vi "VisionExecute.v.vi"   [LabVIEW 2020]
uses:
  <vilib>/Rock Robotics/WPI/ThirdParty/JAS_Junk/TrajLib/Trajectory_Library.lvlib
  <vilib>/Rock Robotics/WPI/ThirdParty/PhotonVisionLib/PhotonVisionLib.lvlib
  <vilib>/Rock Robotics/WPI/ThirdParty/PhotonPoseStrategy_ENUM.ctl
  VisionGlobal.vi
  <vilib>/Rock Robotics/WPI/ThirdParty/JAS_Junk/TrajLib/TypeDef/TRANSLATION2D.ctl
  <vilib>/Rock Robotics/WPI/ThirdParty/JAS_Junk/TrajLib/TypeDef/ROTATION2D.ctl
  <vilib>/Rock Robotics/WPI/ThirdParty/JAS_Junk/TrajLib/TypeDef/POSE2D.ctl
types:
  T1 = typedef "PhotonVisionLib.lvlib/PhotonPoseStrategy_ENUM.ctl" = enum16{"LOWEST_AMBIGUITY", "CLOSEST_TO_CAMERA_HEIGHT", "CLOSEST_TO_REFERENCE_POSE", "CLOSEST_TO_LAST_POSE", "AVERAGE_BEST_TARGETS"}
  T2 = typedef "Trajectory_Library.lvlib/TRANSLATION3D.ctl" = cluster{"X":dbl, "Y":dbl, "Z":dbl}
  T3 = typedef "Trajectory_Library.lvlib/ROTATION3D.ctl" = cluster{"Q_quaternion":T4}
  T4 = typedef "Trajectory_Library.lvlib/QUATERNION.ctl" = cluster{"R":dbl, "V":dbl[]}
  T5 = typedef "Trajectory_Library.lvlib/TRANSFORM3D.ctl" = cluster{"TRANSLATION3D":T2, "ROTATION3D":T3, "XF":bool}
  T6 = typedef "PhotonVisionLib.lvlib/PhotonPipelineResultType.ctl" = cluster{"TargetCount":i32, "Latency_MilliSec":dbl, "Targets":T7[], "TimeStampSec":dbl}
  T7 = typedef "PhotonVisionLib.lvlib/PhotonTrackedTargetType.ctl" = cluster{"Yaw":dbl, "Pitch":dbl, "Area":dbl, "Skew":dbl, "MinAreaRectCorners":T8[], "BestCameraToTarget":T5, "FiiducialId":i32, "AltCameraToTarget":T5, "PoseAmbiguity":dbl, "DetectedCorners":T8[]}
  T8 = typedef "PhotonVisionLib.lvlib/TargetCornerType.ctl" = cluster{"X":dbl, "Y":dbl}
  T9 = typedef "PhotonVisionLib.lvlib/PhotonPoseEstimator_Configuration.ctl" = cluster{"Strategy":T1, "Camera":string, "Initial Pose":T10, "AprilTagField":enum16{"2022 Rapid React", "2023 Charged Up"}, "HighestAmbiguity":dbl, "Use Custom Field":bool, "Custom AprilTag Field":T11, "RobotToCamera":T5}
  T10 = typedef "Trajectory_Library.lvlib/POSE3D.ctl" = cluster{"Translation3d":T2, "Rotation3d":T3}
  T11 = typedef "Trajectory_Library.lvlib/AprilTagFieldLayout.ctl" = cluster{"AprilTagMap":map{i32, T12}, "FieldLength":dbl, "FieldWidth":dbl, "OriginPosition ":T13, "OriginPose3d":T10}
  T12 = typedef "Trajectory_Library.lvlib/AprilTag.ctl" = cluster{"ID":i32, "POSE3D":T10}
  T13 = typedef "Trajectory_Library.lvlib/AprilTagFieldLayoutOrignPosition_ENUM.ctl" = enum16{"kBlueAllianceWallRightSide,", "kRedAllianceWallRightSide,"}
  T14 = typedef "PhotonVisionLib.lvlib/PhotonEstimatedRobotPoseType.ctl" = cluster{"EstimatedPose":T10, "TimeStamp_Seconds":dbl}
  T15 = typedef "Trajectory_Library.lvlib/POSE2D.ctl" = cluster{"TRANSLATION":T16, "ROTATION":T17}
  T16 = typedef "Trajectory_Library.lvlib/TRANSLATION2D.ctl" = cluster{"X":dbl, "Y":dbl}
  T17 = typedef "Trajectory_Library.lvlib/ROTATION2D.ctl" = cluster{"VALUE":dbl, "COS":dbl, "SIN":dbl}
  T18 = typedef "Trajectory_Library.lvlib/SWERVE_DRIVE_KINEMATICS.ctl" = cluster{"NumModules":i32, "InverseKinematics":T19, "ForwardKinematics":T19, "Modules":T16[], "PrevCoR":T16, "SavedModuleStates":T20[]}
  T19 = typedef "NI_Matrix.lvlib/RealMatrix.ctl" = dbl[][]
  T20 = typedef "Trajectory_Library.lvlib/SWERVE_DRIVE_MODULE_STATE.ctl" = cluster{"Speed":dbl, "Angle":T17}
  T21 = typedef "Trajectory_Library.lvlib/SWERVE_DRIVE_MODULE_POSITION.ctl" = cluster{"Distance":dbl, "Angle":T17, "P":bool}
  T22 = typedef "Trajectory_Library.lvlib/SWERVE_DRIVE_POSE_EST2_CONFIG.ctl" = cluster{"Wheel_Locations M":T16[], "Odom X std dev M":dbl, "Odom Y std dev M":dbl, "Odom Heading std dev Rad":dbl, "Vision X std dev M":dbl, "Vision Y std dev M":dbl, "Vision Heading std dev Rad":dbl}
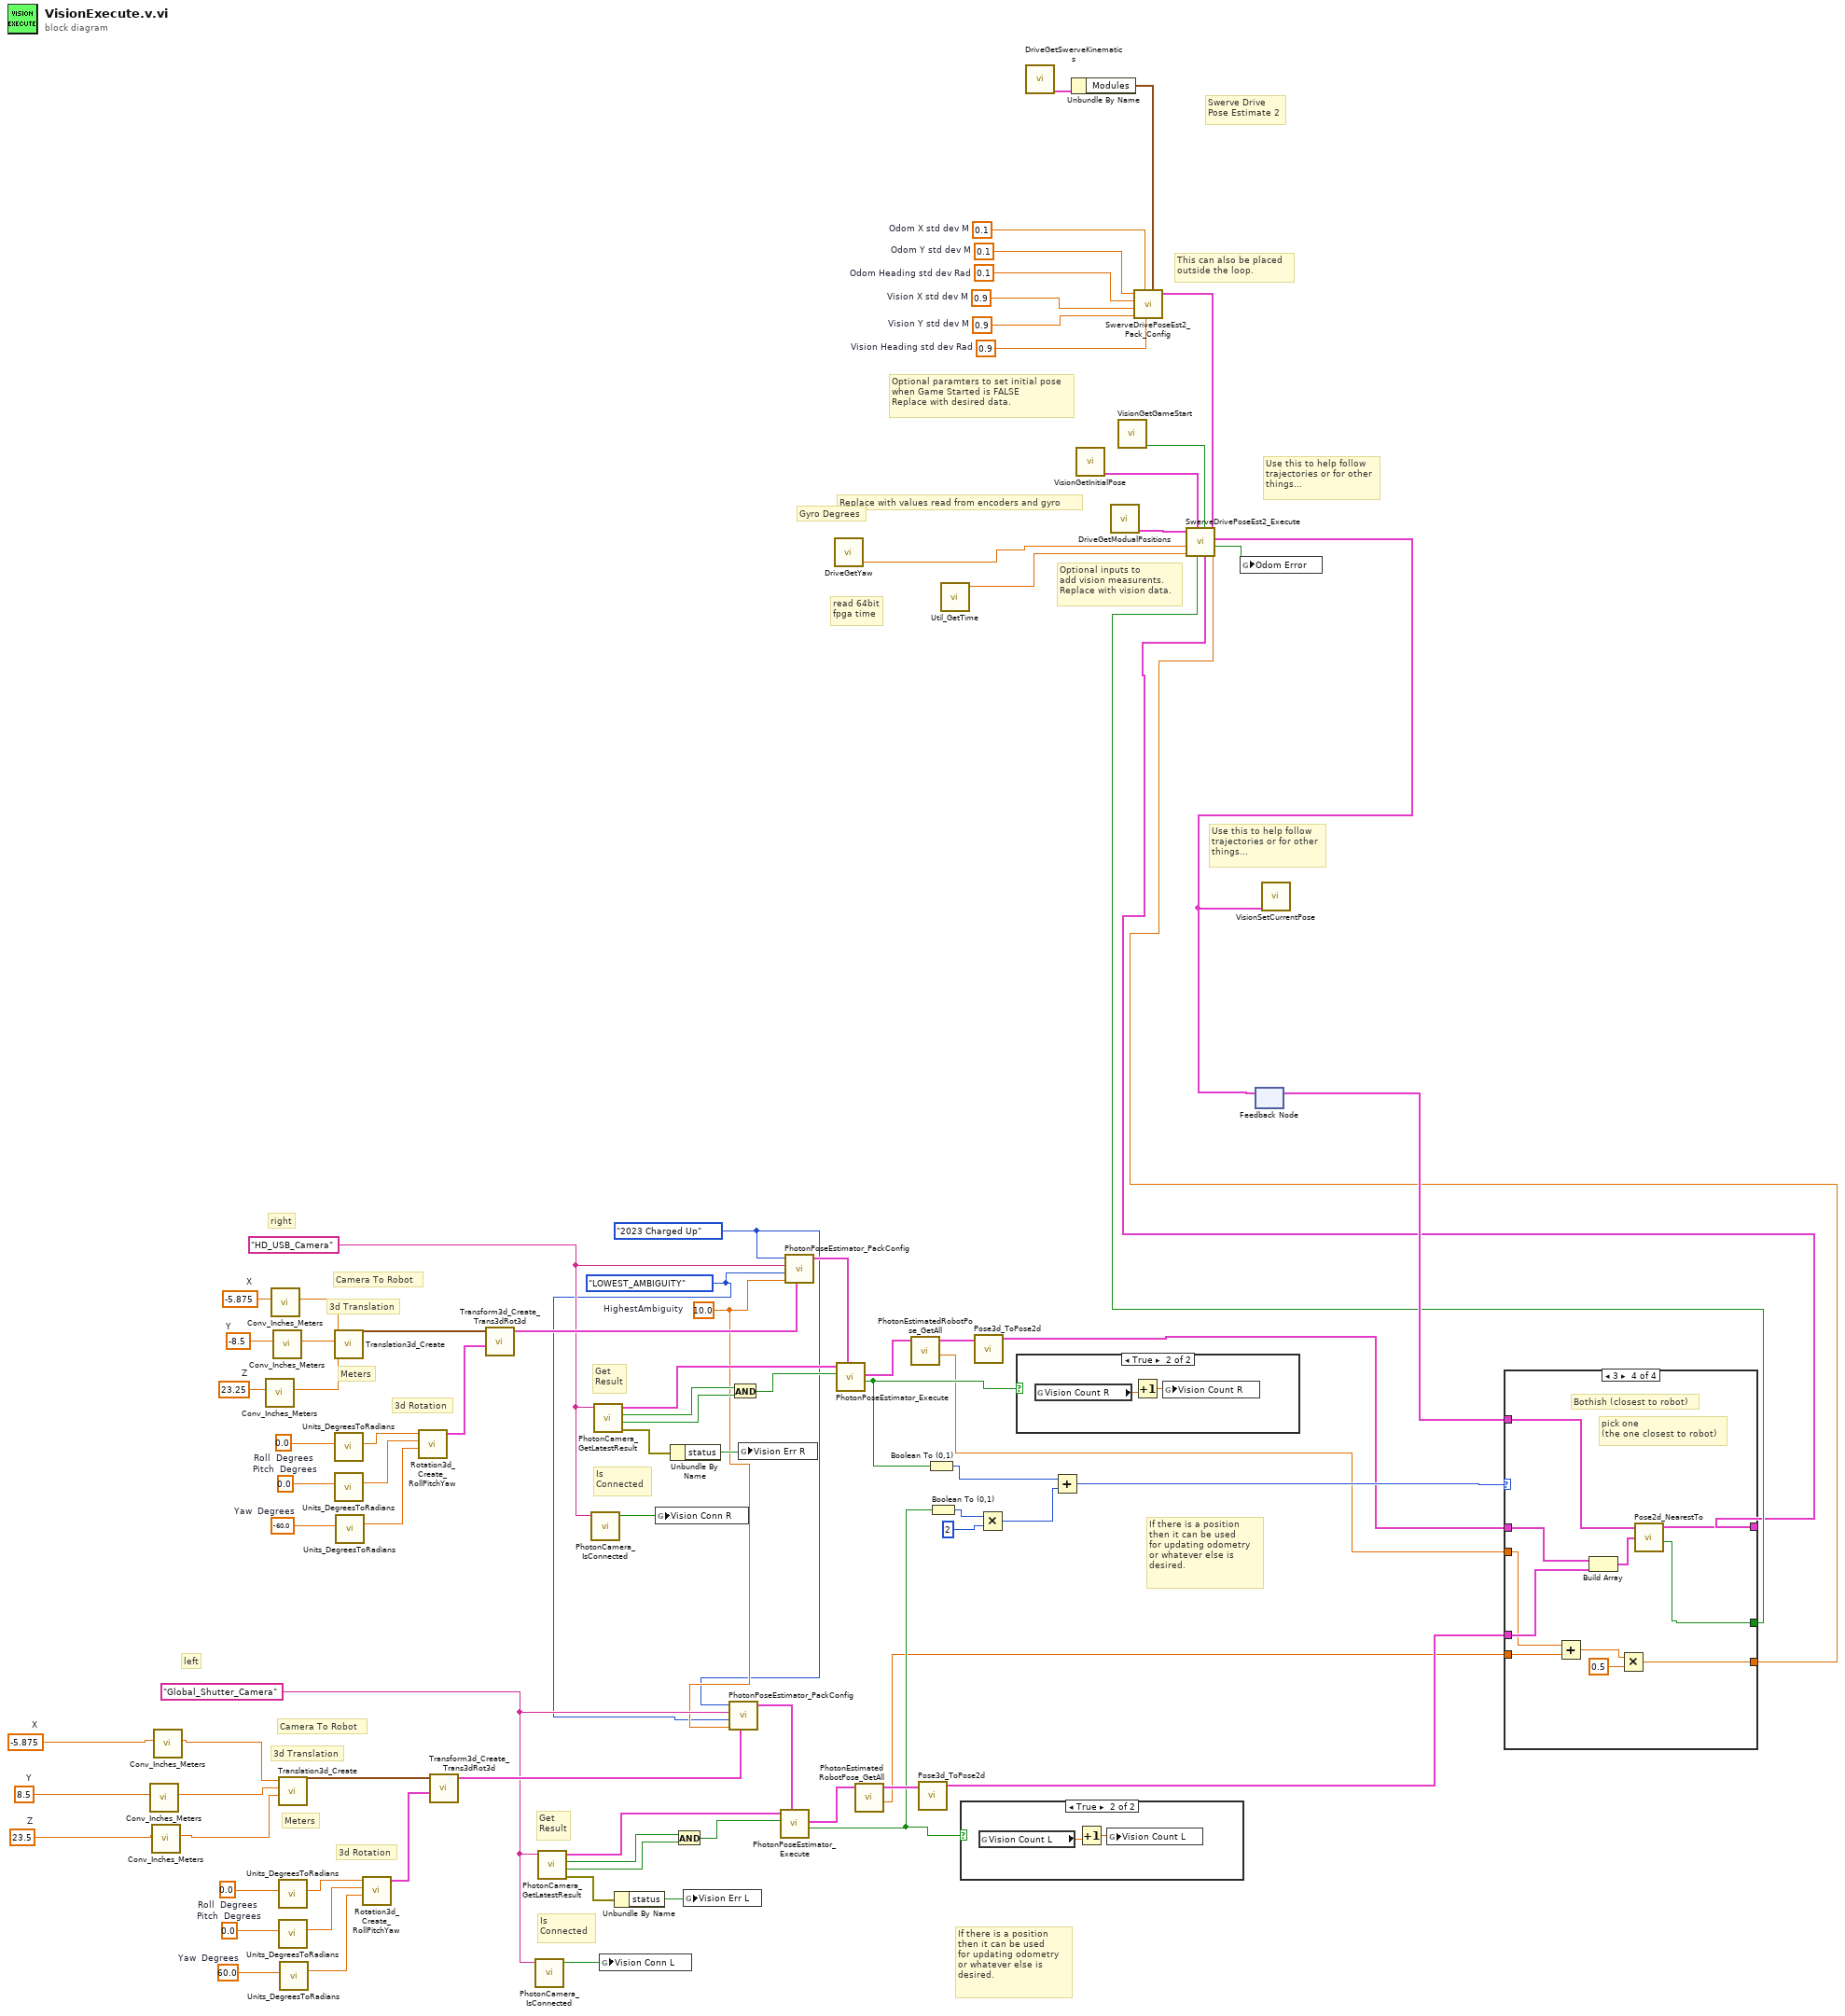
[diagram p0: block diagram]
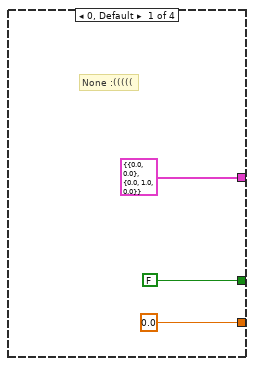
[diagram p2: hidden frame]
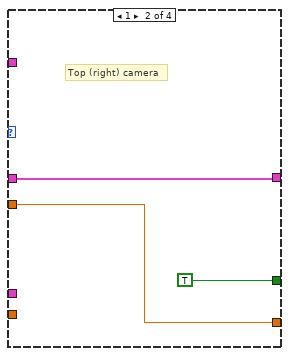
[diagram p3: hidden frame]
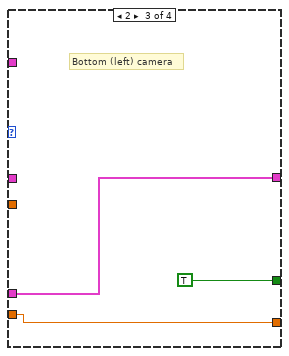
[diagram p4: hidden frame]
diagram:
  w14 = 0.1  # Odom Y std dev M
  w15 = 0.1  # Odom Heading std dev Rad
  w16 = 0.9  # Vision X std dev M
  w17 = 0.9  # Vision Y std dev M
  w18 = 0.1  # Odom X std dev M
  w19 = 0.9  # Vision Heading std dev Rad
  w59 = 0.0  # Roll  Degrees
  w58 = 0.0  # Pitch  Degrees
  w57 = 60.0  # Yaw  Degrees
  w42 = 23.5  # Z
  w46 = -5.875  # X
  w44 = 8.5  # Y
  w53 = "Global_Shutter_Camera" ("CameraName")
  w79 = 0.0  # Roll  Degrees
  w78 = 0.0  # Pitch  Degrees
  w77 = -60.0  # Yaw  Degrees
  w36 = 23.25  # Z
  w40 = -5.875  # X
  w38 = -8.5  # Y
  w34 = 10.0  # HighestAmbiguity
  w33 = PhotonPoseStrategy_ENUM."LOWEST_AMBIGUITY" ("Strategy")
  w32 = enum16{"2022 Rapid React", "2023 Charged Up"}."2023 Charged Up" ("AprilTagField")
  w73 = "HD_USB_Camera" ("CameraName")
  # "Optional inputs to\nadd vision measurents.\nReplace with vision data."
  # "Replace with values read from encoders and gyro"
  # "Optional paramters to set initial pose\nwhen Game Started is FALSE\nReplace with desired data."
  # "read 64bit\nfpga time"
  # "This can also be placed \noutside the loop."
  # "Use this to help follow\ntrajectories or for other\nthings..."
  # "Swerve Drive \nPose Estimate 2"
  # "Use this to help follow\ntrajectories or for other\nthings..."
  # "right"
  # "left"
  # "If there is a position\nthen it can be used\nfor updating odometry\nor whatever else is \ndesired."
  # "Meters"
  # "Camera To Robot"
  # "3d Rotation"
  # "3d Translation"
  # "Is\nConnected"
  # "Get\nResult"
  # "If there is a position\nthen it can be used\nfor updating odometry\nor whatever else is \ndesired."
  # "Meters"
  # "Camera To Robot"
  # "3d Rotation"
  # "3d Translation"
  # "Is\nConnected"
  # "Get\nResult"
  # "Gyro Degrees"
  n1 = call <vilib>:"Conv_Inches_Meters.vi"("INCH"=w44) -> ("Meters"=w43:dbl)  [unwired: 10 in]
  n2 = call <vilib>:"Conv_Inches_Meters.vi"("INCH"=w42) -> ("Meters"=w41:dbl)  [unwired: 10 in]
  n3 = call <vilib>:"Conv_Inches_Meters.vi"("INCH"=w46) -> ("Meters"=w45:dbl)  [unwired: 10 in]
  n4 = call <vilib>:"Conv_Inches_Meters.vi"("INCH"=w36) -> ("Meters"=w35:dbl)  [unwired: 10 in]
  n5 = call <vilib>:"Conv_Inches_Meters.vi"("INCH"=w40) -> ("Meters"=w39:dbl)  [unwired: 10 in]
  n6 = call <vilib>:"Conv_Inches_Meters.vi"("INCH"=w38) -> ("Meters"=w37:dbl)  [unwired: 10 in]
  n7 = call <vilib>:"Translation3d_Create.vi"("Z"=w41, "Y"=w43, "X"=w45) -> ("TRANSLATION3D"=w60:T2)  [unwired: 8 in]
  n8 = call <vilib>:"Units_DegreesToRadians.vi"("Degrees"=w59) -> ("Radians"=w56:dbl)  [unwired: 10 in]
  n9 = call <vilib>:"Units_DegreesToRadians.vi"("Degrees"=w58) -> ("Radians"=w55:dbl)  [unwired: 10 in]
  n10 = call <vilib>:"Units_DegreesToRadians.vi"("Degrees"=w57) -> ("Radians"=w54:dbl)  [unwired: 10 in]
  n11 = call <vilib>:"Translation3d_Create.vi"("Z"=w35, "Y"=w37, "X"=w39) -> ("TRANSLATION3D"=w80:T2)  [unwired: 8 in]
  n12 = call <vilib>:"Units_DegreesToRadians.vi"("Degrees"=w79) -> ("Radians"=w76:dbl)  [unwired: 10 in]
  n13 = call <vilib>:"Units_DegreesToRadians.vi"("Degrees"=w78) -> ("Radians"=w75:dbl)  [unwired: 10 in]
  n14 = call <vilib>:"Units_DegreesToRadians.vi"("Degrees"=w77) -> ("Radians"=w74:dbl)  [unwired: 10 in]
  n15 = call <vilib>:"Rotation3d_Create_RollPitchYaw.vi"("Yaw"=w54, "Pitch"=w55, "Roll"=w56) -> ("Rotation3d"=w61:T3)  [unwired: 8 in]
  n16 = call <vilib>:"Rotation3d_Create_RollPitchYaw.vi"("Yaw"=w74, "Pitch"=w75, "Roll"=w76) -> ("Rotation3d"=w81:T3)  [unwired: 8 in]
  n17 = call <vilib>:"Transform3d_Create_Trans3dRot3d.vi"("Rotation3d"=w61, "Translation3d"=w60) -> ("Transform3d"=w62:T5)  [unwired: 9 in]
  n18 = call <vilib>:"Transform3d_Create_Trans3dRot3d.vi"("Rotation3d"=w81, "Translation3d"=w80) -> ("Transform3d"=w82:T5)  [unwired: 9 in]
  n19 = call <vilib>:"PhotonCamera_IsConnected.vi"("CameraName"=w53) -> ("IsConnected"=w49:bool)  [unwired: 9 in, 1 out]
  n20 = call <vilib>:"PhotonCamera_GetLatestResult.vi"("CameraName"=w53) -> ("error out"=w48:errorcluster, "New Data"=w66:bool, "HasTargets"=w65:bool, "PipelineResult"=w63:T6)  [unwired: 7 in]
  n21 = call <vilib>:"PhotonCamera_IsConnected.vi"("CameraName"=w73) -> ("IsConnected"=w69:bool)  [unwired: 9 in, 1 out]
  n22 = call <vilib>:"PhotonCamera_GetLatestResult.vi"("CameraName"=w73) -> ("error out"=w68:errorcluster, "New Data"=w86:bool, "HasTargets"=w85:bool, "PipelineResult"=w83:T6)  [unwired: 7 in]
  n23 = global write "VisionGlobal.vi" "Vision Conn L"(w49) -> ()
  n24 = Unbundle By Name(w48) -> ("status"=w47:bool)
  n25 = global write "VisionGlobal.vi" "Vision Conn R"(w69) -> ()
  n26 = Unbundle By Name(w68) -> ("status"=w67:bool)
  n27 = And(x=w65, y=w66) -> (x .and. y?=w64:bool)
  n28 = global write "VisionGlobal.vi" "Vision Err L"(w47) -> ()
  n29 = call <vilib>:"PhotonPoseEstimator_PackConfig.vi"("RobotToCamera"=w62, "HighestAmbiguity"=w34, "Strategy"=w33, "Camera"=w53, "AprilTagField"=w32) -> ("PoseEstimator_Configuration"=w52:T9)  [unwired: 6 in]
  n30 = And(x=w85, y=w86) -> (x .and. y?=w84:bool)
  n31 = global write "VisionGlobal.vi" "Vision Err R"(w67) -> ()
  n32 = call <vilib>:"PhotonPoseEstimator_Execute.vi"("Configuration"=w52, "PIpeline Has \nNew Results"=w64, "PipelineResult"=w63) -> ("Pos Found"=w30:bool, "PhotonEstimatedRobotPose"=w51:T14)  [unwired: 6 in, 1 out]
  n33 = call <vilib>:"PhotonPoseEstimator_PackConfig.vi"("RobotToCamera"=w82, "HighestAmbiguity"=w34, "Strategy"=w33, "Camera"=w73, "AprilTagField"=w32) -> ("PoseEstimator_Configuration"=w72:T9)  [unwired: 6 in]
  n34 = call "DriveGetYaw.vi"() -> ("Yaw"=w9:dbl)  [unwired: 11 in]
  n35 = call <vilib>:"PhotonPoseEstimator_Execute.vi"("Configuration"=w72, "PIpeline Has \nNew Results"=w84, "PipelineResult"=w83) -> ("Pos Found"=w31:bool, "PhotonEstimatedRobotPose"=w71:T14)  [unwired: 6 in, 1 out]
  n36 = call <vilib>:"PhotonEstimatedRobotPose_GetAll.vi"("PhotonEstimatedRobotPose"=w51) -> ("TimeStamp_Seconds"=w20:dbl, "EstimatedPose"=w50:T10)  [unwired: 9 in]
  n37 = call <vilib>:"PhotonEstimatedRobotPose_GetAll.vi"("PhotonEstimatedRobotPose"=w71) -> ("TimeStamp_Seconds"=w21:dbl, "EstimatedPose"=w70:T10)  [unwired: 9 in]
  n38 = call <vilib>:"Pose3d_ToPose2d.vi"("in Pose3d"=w50) -> ("out Pose2d"=w23:T15)  [unwired: 10 in]
  n39 = Boolean To (0,1)(Boolean=w31) -> (0, 1=w26:i16)
  n40 = Boolean To (0,1)(Boolean=w30) -> (0, 1=w29:i16)
  n41 = call <vilib>:"Util_GetTime.vi"() -> ("FPGA_Time_Seconds"=w6:dbl)  [unwired: 9 in, 2 out]
  n42 = case shown="True" w30 {
    frame False {
    }
    frame True {
      n43 = global read "VisionGlobal.vi" "Vision Count L"() -> (w87:dbl)
      n44 = Increment(x=w87) -> (x+1=w88:dbl)
      n45 = global write "VisionGlobal.vi" "Vision Count L"(w88) -> ()
    }
  }
  n46 = call <vilib>:"Pose3d_ToPose2d.vi"("in Pose3d"=w70) -> ("out Pose2d"=w24:T15)  [unwired: 10 in]
  n47 = Multiply(x=w29, y=i16 2) -> (x*y=w27:i16)
  n48 = case shown="True" w31 {
    frame False {
    }
    frame True {
      n49 = global read "VisionGlobal.vi" "Vision Count R"() -> (w89:dbl)
      n50 = Increment(x=w89) -> (x+1=w90:dbl)
      n51 = global write "VisionGlobal.vi" "Vision Count R"(w90) -> ()
    }
  }
  n52 = call "DriveGetSwerveKinematics.vi"() -> ("SWERVE_DRIVE_KINEMATICS"=w2:T18)  [unwired: 11 in]
  n53 = Add(x=w26, y=w27) -> (x+y=w25:i16)
  n54 = Unbundle By Name(w2) -> ("Modules"=w1:T16[])
  n55 = call "VisionGetInitialPose.vi"() -> ("InitialPose"=w7:T15)  [unwired: 10 in]
  n56 = call "DriveGetModualPositions.vi"() -> ("Swerve_Drive_Modual_Position"=w10:T21[])  [unwired: 11 in]
  n57 = call "VisionGetGameStart.vi"() -> ("Game Start"=w8:bool)  [unwired: 11 in]
  n58 = call <vilib>:"SwerveDrivePoseEst2_Pack_Config.vi"("Wheel_Locations M"=w1, "Vision Heading std dev Rad"=w19, "Odom X std dev M"=w18, "Vision Y std dev M"=w17, "Vision X std dev M"=w16, "Odom Heading std dev Rad"=w15, "Odom Y std dev M"=w14) -> ("SwervePoseEst2Config"=w13:T22)  [unwired: 4 in]
  n59 = feedback #1() -> (w22:T15)  [unwired: 1 in]
  n60 = case shown="3" w25 {
    tunnel: w24 -> [_ w95 _ w108]
    tunnel: w23 -> [_ _ w98 w107]
    tunnel: w22 -> [_ _ _ w109]
    tunnel: [FALSE ("Found") TRUE ("Found") TRUE ("Found") w105] -> w5
    tunnel: w21 -> [_ w96 _ w104]
    tunnel: w20 -> [_ _ w99 w103]
    tunnel: [T15 {"TRANSLATION"={"X"=0.0, "Y"=0.0}, "ROTATION"={"VALUE"=0.0, "COS"=1.0, "SIN"=0.0}} ("Nearest Pose") w95 w98 w106] -> w4
    tunnel: [0.0 w96 w99 w100] -> w3
    frame 0, Default {
      # "None :((((("
    }
    frame 1 {
      # "Top (right) camera"
    }
    frame 2 {
      # "Bottom (left) camera"
    }
    frame 3 {
      # "pick one \n(the one closest to robot)"
      # "Bothish (closest to robot)"
      n61 = Add(x=w104, y=w103) -> (x+y=w102:dbl)
      n62 = Build Array(w108, w107) -> (w110:T15[])
      n63 = Multiply(x=w102, y=0.5) -> (x*y=w100:dbl)
      n64 = call <vilib>:"Pose2d_NearestTo.vi"("other POSE"=w110, "in POSE"=w109) -> ("Found"=w105:bool, "Nearest Pose"=w106:T15)  [unwired: 8 in]
    }
  }
  n65 = call <vilib>:"SwerveDrivePoseEst2_Execute.vi"("Vision TImeStamp_Seconds"=w3, "SwervePoseEst2Config"=w13, "visionRobotPose"=w4, "Game Started"=w8, "Add Vision Meas"=w5, "InitialPose"=w7, "Pass Through Time"=w6, "Gyro Degrees"=w9, "Module Positions"=w10) -> ("Error"=w11:bool, "Estimated Pose"=w12:T15)  [unwired: 1 in]
  n66 = global write "VisionGlobal.vi" "Odom Error"(w11) -> ()
  n67 = feedback-in #1(w12) -> ()
  n68 = call "VisionSetCurrentPose.vi"("Current Pose"=w12) -> ()  [unwired: 11 in]
